vi "err_id.vi"() -> (0 "error code":i32=6998)   [LabVIEW 2019]
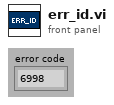
[diagram p1: front panel]
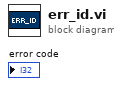
[diagram p0: block diagram]
diagram:
